vi "总磷总氮断电保存全局变量.vi"() -> ()   [LabVIEW 2016, in "斯坦道总氮.lvlib"]
panel:
  in  "吸光度":sgl
  in  "协议":u16(ring)=1 items=["斯坦道协议"=1, "国标协议"=2]
  in  "波特率":u32(ring)=115200 items=["115200"=115200, "9600"=9600]
  out "CODmn消解时长":dbl=30.0 caption="消解时长："
  in  "CODMn自动测试量程配置":T1={"水样测试量程模式"=enum."AUTO", "空白核查量程模式"=enum."AUTO", "跨度核查量程模式"=enum."AUTO", "加标回收量程模式"=enum."AUTO", "标样核查量程模式"=enum."AUTO"}
  in  "氟化物自动测试量程配置":T1={"水样测试量程模式"=enum."AUTO", "空白核查量程模式"=enum."AUTO", "跨度核查量程模式"=enum."AUTO", "加标回收量程模式"=enum."AUTO", "标样核查量程模式"=enum."AUTO"}
  in  "标样核查自动补测":bool caption="通讯连接"
  in  "跨度核查自动补测":bool caption="通讯连接"
  in  "零点核查自动补测":bool caption="通讯连接"
  in  "低量程上限":T2={"总磷"=1.0, "总氮"=10.0, "氨氮"=1.0, "磷酸盐"=1.0, "硝氮"=2.0, "亚硝氮"=0.6, "硅酸盐"=5.0, "硫化物"=2.0, "COD"=200.0, "氟化物"=1.5, "CODMn"=10.0}
  out "校准条件":cluster{"线性相关系数":dbl}={"线性相关系数"=0.99}
  in  "简易流程路径":path=path "流程.xml"
  out "CODcr消解时长":dbl=30.0 caption="消解时长："
  out "总氮消解时长":dbl=30.0 caption="消解时长："
  out "总磷消解时长":dbl=30.0 caption="消解时长："
  in  "盐度自动补偿：":bool
  in  "阀口名称":T3={"V"="试剂1", "V 2"="试剂2", "V 3"="试剂3", "V 4"="试剂4", "V 5"="试剂5", "V 6"="试剂6", "V 7"="试剂7", "V 8"="试剂8", "V 9"="试剂9", "V 10"="试剂10", "V 11"="试剂11", "V 12"="试剂12", "V9-1"="试剂13", "V9-2"="试剂14"}
  in  "硫化物自动测试量程配置":T1={"水样测试量程模式"=enum."AUTO", "空白核查量程模式"=enum."AUTO", "跨度核查量程模式"=enum."AUTO", "加标回收量程模式"=enum."AUTO", "标样核查量程模式"=enum."AUTO"}
  in  "硅酸盐自动测试量程配置":T1={"水样测试量程模式"=enum."AUTO", "空白核查量程模式"=enum."AUTO", "跨度核查量程模式"=enum."AUTO", "加标回收量程模式"=enum."AUTO", "标样核查量程模式"=enum."AUTO"}
  in  "亚硝氮自动测试量程配置":T1={"水样测试量程模式"=enum."AUTO", "空白核查量程模式"=enum."AUTO", "跨度核查量程模式"=enum."AUTO", "加标回收量程模式"=enum."AUTO", "标样核查量程模式"=enum."AUTO"}
  in  "硝氮自动测试量程配置":T1={"水样测试量程模式"=enum."AUTO", "空白核查量程模式"=enum."AUTO", "跨度核查量程模式"=enum."AUTO", "加标回收量程模式"=enum."AUTO", "标样核查量程模式"=enum."AUTO"}
  in  "磷酸盐自动测试量程配置":T1={"水样测试量程模式"=enum."AUTO", "空白核查量程模式"=enum."AUTO", "跨度核查量程模式"=enum."AUTO", "加标回收量程模式"=enum."AUTO", "标样核查量程模式"=enum."AUTO"}
  in  "氨氮自动测试量程配置":T1={"水样测试量程模式"=enum."AUTO", "空白核查量程模式"=enum."AUTO", "跨度核查量程模式"=enum."AUTO", "加标回收量程模式"=enum."AUTO", "标样核查量程模式"=enum."AUTO"}
  in  "COD自动测试量程配置":T1={"水样测试量程模式"=enum."AUTO", "空白核查量程模式"=enum."AUTO", "跨度核查量程模式"=enum."AUTO", "加标回收量程模式"=enum."AUTO", "标样核查量程模式"=enum."AUTO"}
  in  "MB通信方式选择":enum16{"串口", "TCP"}(ring)
  in  "PORT":string="502"
  in  "IP":string
  in  "VISA Resource":refnum<visa-resource-name>
  in  "运行周期":T4={"运行模式"=enum."维护模式", "质控频次"=enum."关闭", "空白核查时间"=2, "跨度核查时间"=6, "测量间隔"=240} {"跨度核查时间" items=["00H", "01H", "02H", "03H", "04H", "05H", "06H", "07H", "08H", "09H", "10H", "11H", "12H", "13H", "14H", "15H", "16H", "17H", "18H", "19H", "20H", "21H", "22H", "23H", "关闭"]; "空白核查时间" items=["00H", "01H", "02H", "03H", "04H", "05H", "06H", "07H", "08H", "09H", "10H", "11H", "12H", "13H", "14H", "15H", "16H", "17H", "18H", "19H", "20H", "21H", "22H", "23H", "关闭"]}
  in  "流程路径":path=path "data/流程.xml"
  in  "总氮自动测试量程配置":T1={"水样测试量程模式"=enum."AUTO", "空白核查量程模式"=enum."AUTO", "跨度核查量程模式"=enum."AUTO", "加标回收量程模式"=enum."AUTO", "标样核查量程模式"=enum."AUTO"}
  in  "质控参数设置":T5 {"CODMn标准液标准偏差" format="%#_g%"; "CODMn跨度标准液偏差" format="%#_g%"; "氟化物标准液标准偏差" format="%#_g%"; "氟化物跨度标准液偏差" format="%#_g%"; "硅酸盐标准液标准偏差" format="%#_g%"; "硅酸盐跨度标准液偏差" format="%#_g%"; "硫化物标准液标准偏差" format="%#_g%"; "硫化物跨度标准液偏差" format="%#_g%"; "亚硝氮标准液标准偏差" format="%#_g%"; "亚硝氮跨度标准液偏差" format="%#_g%"; "硝氮标准液标准偏差" format="%#_g%"; "硝氮跨度标准液偏差" format="%#_g%"; "磷酸盐标准液标准偏差" format="%#_g%"; "磷酸盐跨度标准液偏差" format="%#_g%"; "氨氮标准液标准偏差" format="%#_g%"; "氨氮跨度标准液偏差" format="%#_g%"; "COD标准液标准偏差" format="%#_g%"; "COD跨度标准液偏差" format="%#_g%"; "总氮标准液标准偏差" format="%#_g%"; "总氮跨度标准液偏差" format="%#_g%"; "总磷标准液标准偏差" format="%#_g%"; "总磷跨度标准液偏差" format="%#_g%"}
  in  "总磷自动测试量程配置":T1={"水样测试量程模式"=enum."AUTO", "空白核查量程模式"=enum."AUTO", "跨度核查量程模式"=enum."AUTO", "加标回收量程模式"=enum."AUTO", "标样核查量程模式"=enum."AUTO"}
  # "min"
  # "min"
  # "min"
  # "min"
  # "运行模式："
  # "质控频次："
  # "零点核查时间："
  # "跨度核查时间："
  # "测量间隔："
  # "质控参数设置"
  # "总氮"
  # "COD"
  # "氨氮"
  # "磷酸盐"
  # "硝氮"
  # "亚硝氮"
  # "硫化物"
  # "硅酸盐"
  # "监测参数"
  # "总磷"
  # "氟化物"
  # "CODMn"
  # "跨度值"
  # "零点核查标准液浓度"
  # "跨度核查标准液浓度"
  # "标样核查标准液浓度"
  # "零点核查标准液偏差"
  # "跨度核查标准液偏差"
  # "标样核查标准液偏差"
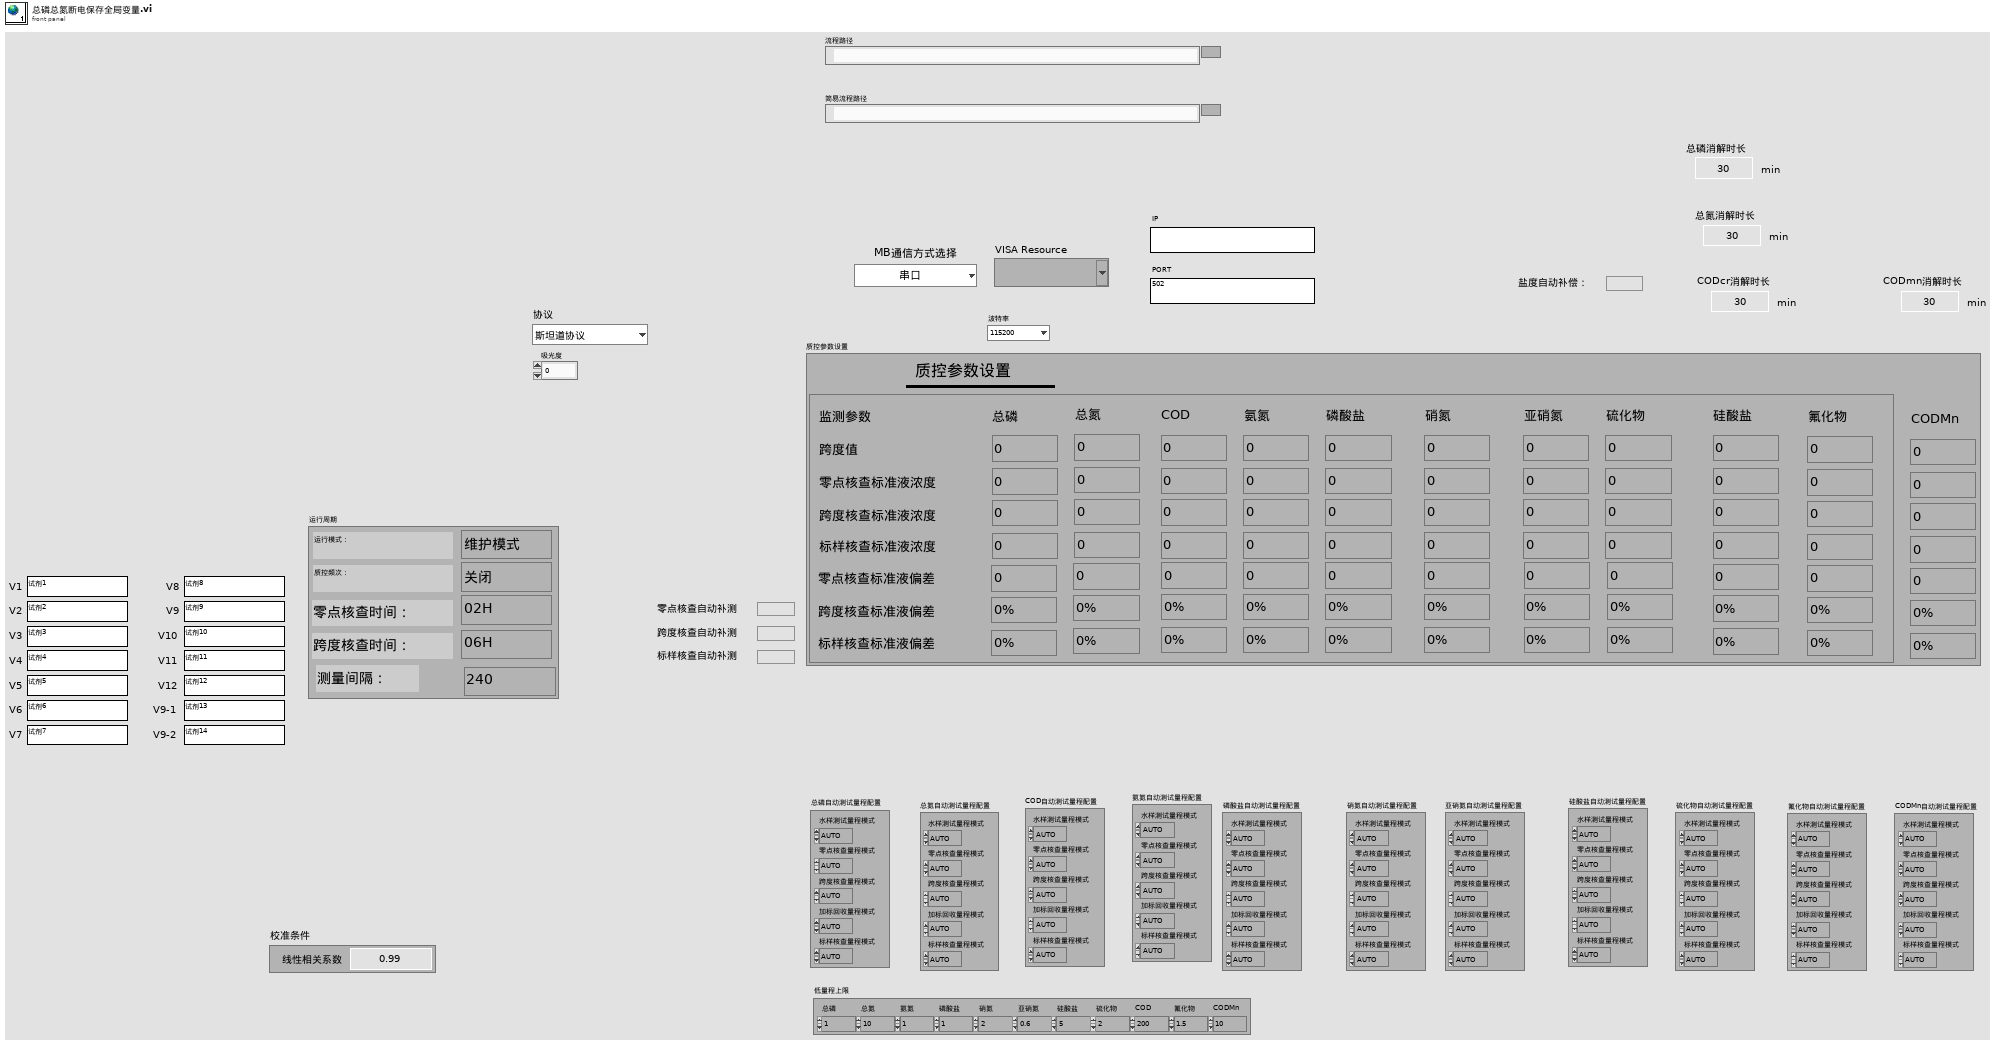
[diagram p1: front panel]
types:
  T1 = cluster{"水样测试量程模式":enum16{"H", "L", "AUTO"}, "空白核查量程模式":enum16{"H", "L", "AUTO"}, "跨度核查量程模式":enum16{"H", "L", "AUTO"}, "加标回收量程模式":enum16{"H", "L", "AUTO"}, "标样核查量程模式":enum16{"H", "L", "AUTO"}}
  T2 = cluster{"总磷":dbl, "总氮":dbl, "氨氮":dbl, "磷酸盐":dbl, "硝氮":dbl, "亚硝氮":dbl, "硅酸盐":dbl, "硫化物":dbl, "COD":dbl, "氟化物":dbl, "CODMn":dbl}
  T3 = cluster{"V":string, "V 2":string, "V 3":string, "V 4":string, "V 5":string, "V 6":string, "V 7":string, "V 8":string, "V 9":string, "V 10":string, "V 11":string, "V 12":string, "V9-1":string, "V9-2":string}
  T4 = cluster{"运行模式":enum16{"维护模式", "常规模式", "应急模式", "质控模式", "性能测试"}, "质控频次":enum16{"关闭", "每天", "星期一", "星期二", "星期三", "星期四", "星期五", "星期六", "星期日"}, "空白核查时间":u16, "跨度核查时间":u16, "测量间隔":u16}
  T5 = cluster{"总磷跨度值":dbl, "总磷零点标准液浓度":dbl, "总磷跨度标准液浓度":dbl, "总磷标准液标准浓度":dbl, "总氮跨度值":dbl, "总氮零点标准液浓度":dbl, "总氮跨度标准液浓度":dbl, "总氮标准液标准浓度":dbl, "COD跨度值":dbl, "COD零点标准液浓度":dbl, "COD跨度标准液浓度":dbl, "COD标准液标准浓度":dbl, "氨氮跨度值":dbl, "氨氮零点标准液浓度":dbl, "氨氮跨度标准液浓度":dbl, "氨氮标准液标准浓度":dbl, "磷酸盐跨度值":dbl, "磷酸盐零点标准液浓度":dbl, "磷酸盐跨度标准液浓度":dbl, "磷酸盐标准液标准浓度":dbl, "硝氮跨度值":dbl, "硝氮零点标准液浓度":dbl, "硝氮跨度标准液浓度":dbl, "硝氮标准液标准浓度":dbl, "亚硝氮跨度值":dbl, "亚硝氮零点标准液浓度":dbl, "亚硝氮跨度标准液浓度":dbl, "亚硝氮标准液标准浓度":dbl, "硫化物跨度值":dbl, "硫化物零点标准液浓度":dbl, "硫化物跨度标准液浓度":dbl, "硫化物标准液标准浓度":dbl, "硅酸盐跨度值":dbl, "硅酸盐零点标准液浓度":dbl, "硅酸盐跨度标准液浓度":dbl, "硅酸盐标准液标准浓度":dbl, "总磷零点标准液偏差":dbl, "总磷跨度标准液偏差":dbl, "总磷标准液标准偏差":dbl, "总氮零点标准液偏差":dbl, "总氮跨度标准液偏差":dbl, "总氮标准液标准偏差":dbl, "COD零点标准液偏差":dbl, "COD跨度标准液偏差":dbl, "COD标准液标准偏差":dbl, "氨氮零点标准液偏差":dbl, "氨氮跨度标准液偏差":dbl, "氨氮标准液标准偏差":dbl, "磷酸盐零点标准液偏差":dbl, "磷酸盐跨度标准液偏差":dbl, "磷酸盐标准液标准偏差":dbl, "硝氮零点标准液偏差":dbl, "硝氮跨度标准液偏差":dbl, "硝氮标准液标准偏差":dbl, "亚硝氮零点标准液偏差":dbl, "亚硝氮跨度标准液偏差":dbl, "亚硝氮标准液标准偏差":dbl, "硫化物零点标准液偏差":dbl, "硫化物跨度标准液偏差":dbl, "硫化物标准液标准偏差":dbl, "硅酸盐零点标准液偏差":dbl, "硅酸盐跨度标准液偏差":dbl, "硅酸盐标准液标准偏差":dbl, "氟化物跨度值":dbl, "氟化物零点标准液浓度":dbl, "氟化物跨度标准液浓度":dbl, "氟化物标准液标准浓度":dbl, "氟化物零点标准液偏差":dbl, "氟化物跨度标准液偏差":dbl, "氟化物标准液标准偏差":dbl, "CODMn跨度值":dbl, "CODMn零点标准液浓度":dbl, "CODMn跨度标准液浓度":dbl, "CODMn标准液标准浓度":dbl, "CODMn零点标准液偏差":dbl, "CODMn跨度标准液偏差":dbl, "CODMn标准液标准偏差":dbl}
diagram:
